vi "BackupOldFileCreatNewFile.vi"(8 "error in":errorcluster, 10 "Data In":variant, 11 "Path":path=path "D:/123/data") -> (0 "error out":errorcluster)   [LabVIEW 2015]
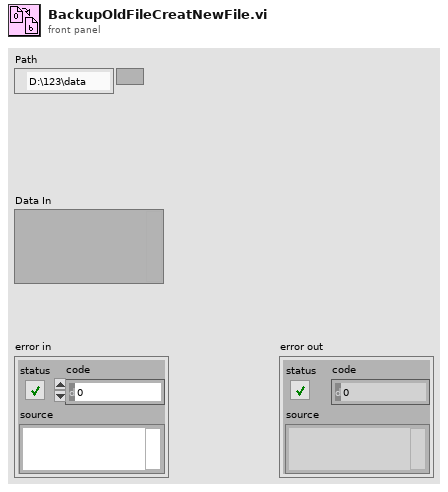
[diagram p1: front panel]
types:
  T1 = enum16{"open", "replace", "create", "open or create", "replace or create", "replace or create with confirmation"}
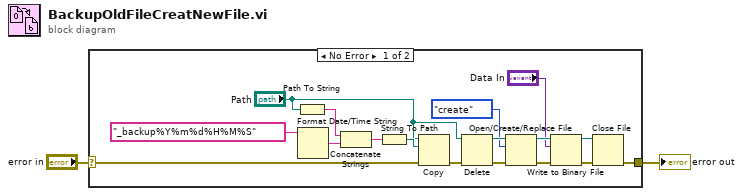
[diagram p0: block diagram]
diagram:
  n1 = case shown="No Error" "error in" {
    selector: "error in" -> [w4 w20]
    tunnel: [w3 w20] -> w1
    frame No Error {
      n2 = Path To String(path="Path") -> (string=w18:string)
      n3 = Format Date/Time String(time format string (%c)="_backup%Y%m%d%H%M%S") -> (date/time string=w17:string)  [unwired: 2 in]
      n4 = Concatenate Strings(w18, w17) -> (w16:string)
      n5 = String To Path(string=w16) -> (path=w15:path)
      n6 = Copy(8:w4, 10:w15, 11:"Path") -> (0:w13:errorcluster)  [unwired: 2 in, 2 out]
      n7 = Delete(path (use dialog)="Path", error in=w13) -> (deleted path=w12:path, error out=w11:errorcluster)  [unwired: 3 in, 1 out]
      n8 = Open/Create/Replace File(file path (use dialog)=w12, error in=w11, operation (0:open)=T1."create") -> (refnum out=w9:refnum<file>, error out=w7:errorcluster)  [unwired: 3 in, 1 out]
      n9 = Write to Binary File(file (use dialog)=w9, data="Data In", error in=w7) -> (refnum out=w8:refnum<file>, error out=w6:errorcluster)  [unwired: 3 in, 1 out]
      n10 = Close File(refnum=w8, error in=w6) -> (error out=w3:errorcluster)  [unwired: 1 out]
    }
    frame Error {
    }
  }
  "error out" <- w1
